vi "RPC Method RouteGuide GetFeature.vi"(3 "error in (no error)":errorcluster, 4 "gRPCid in":T2, 5 "DNL_LabVIEW Object in":refnum<class "RouteGuideImpl.lvclass">) -> (0 "error out":errorcluster, 1 "gRPCid out":T2, 2 "DNL_LabVIEW Object out":refnum<class "RouteGuideImpl.lvclass">)   [LabVIEW 2019, in "UserCode_impl_server.lvlib" / "RouteGuideImpl.lvclass"]
uses:
  RouteGuideImpl.lvclass
  <vilib>/gRPC/LabVIEW gRPC Library/Shared/grpcId.ctl
  Generated_stub_server/RPC Messages/routeguide_Point.ctl
  Generated_stub_server/RPC Service/RouteGuideStub/RouteGuideStub.lvclass
  Generated_stub_server/Generated_stub_server.lvlib
  <vilib>/gRPC/LabVIEW gRPC Library/grpc-lvsupport-release.lvlib
panel:
  in  "?":cluster{"name":string, "location":T1}
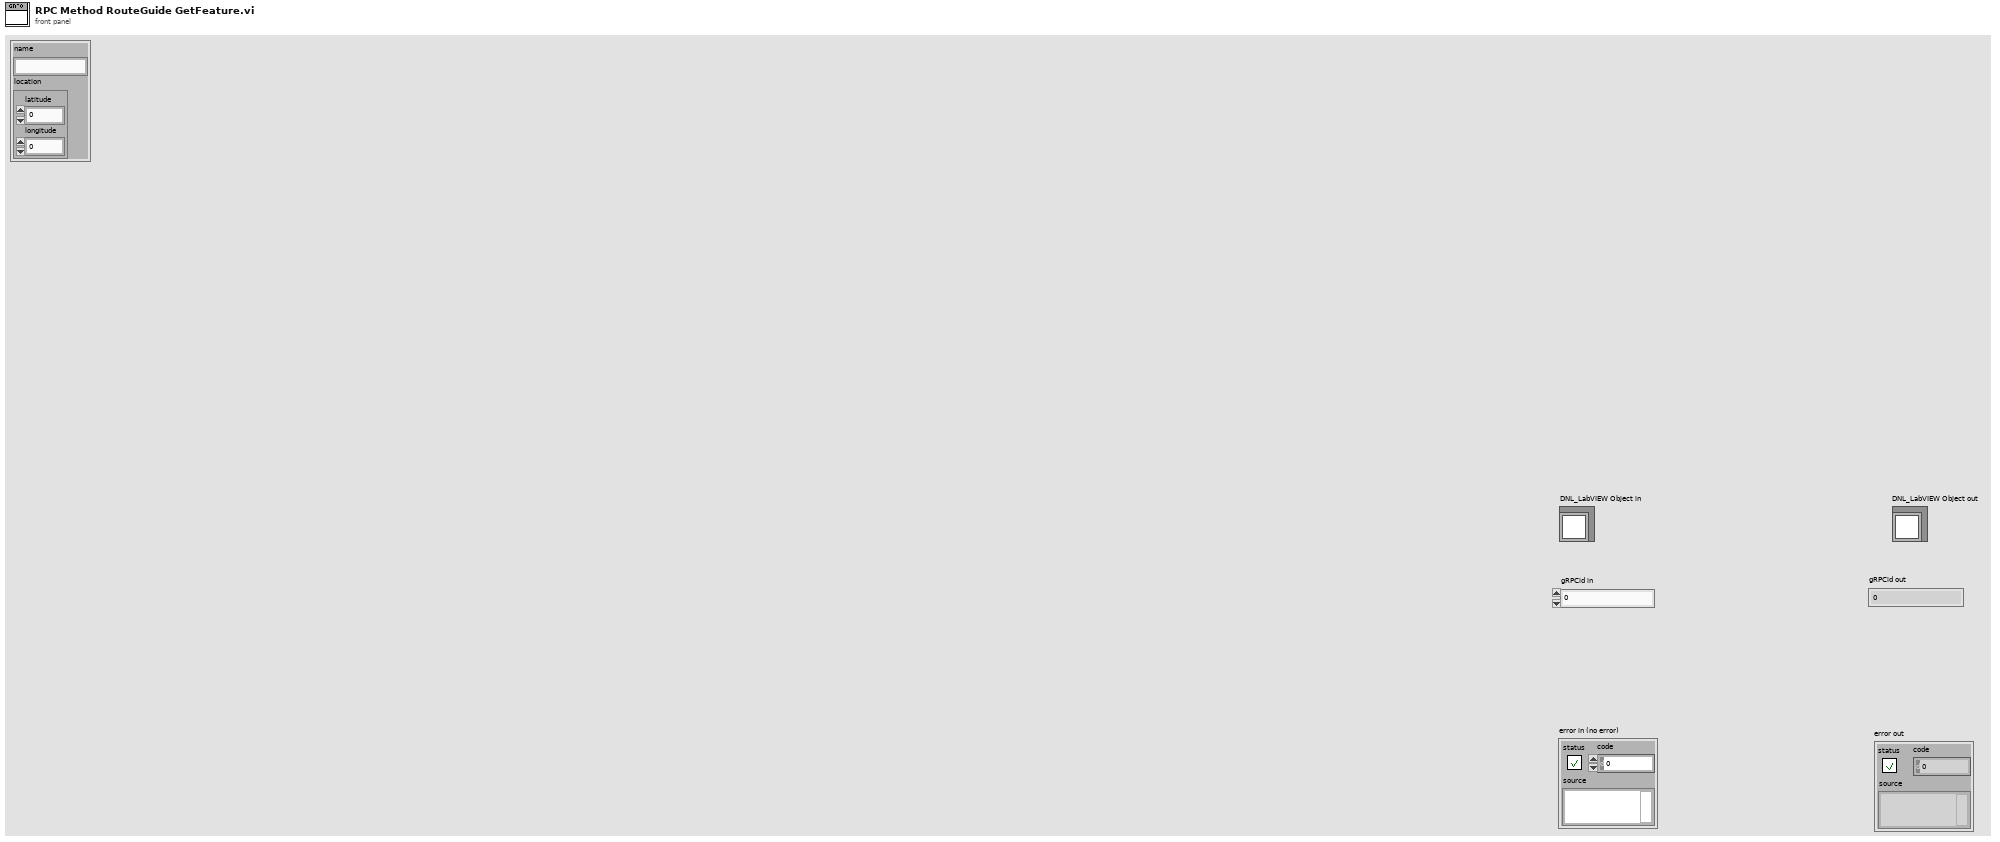
[diagram p1: front panel]
types:
  T1 = typedef "Generated_stub_server.lvlib/routeguide_Point.ctl" = cluster{"latitude":i32, "longitude":i32}
  T2 = typedef "grpc-lvsupport-release.lvlib/grpcId.ctl" = u64
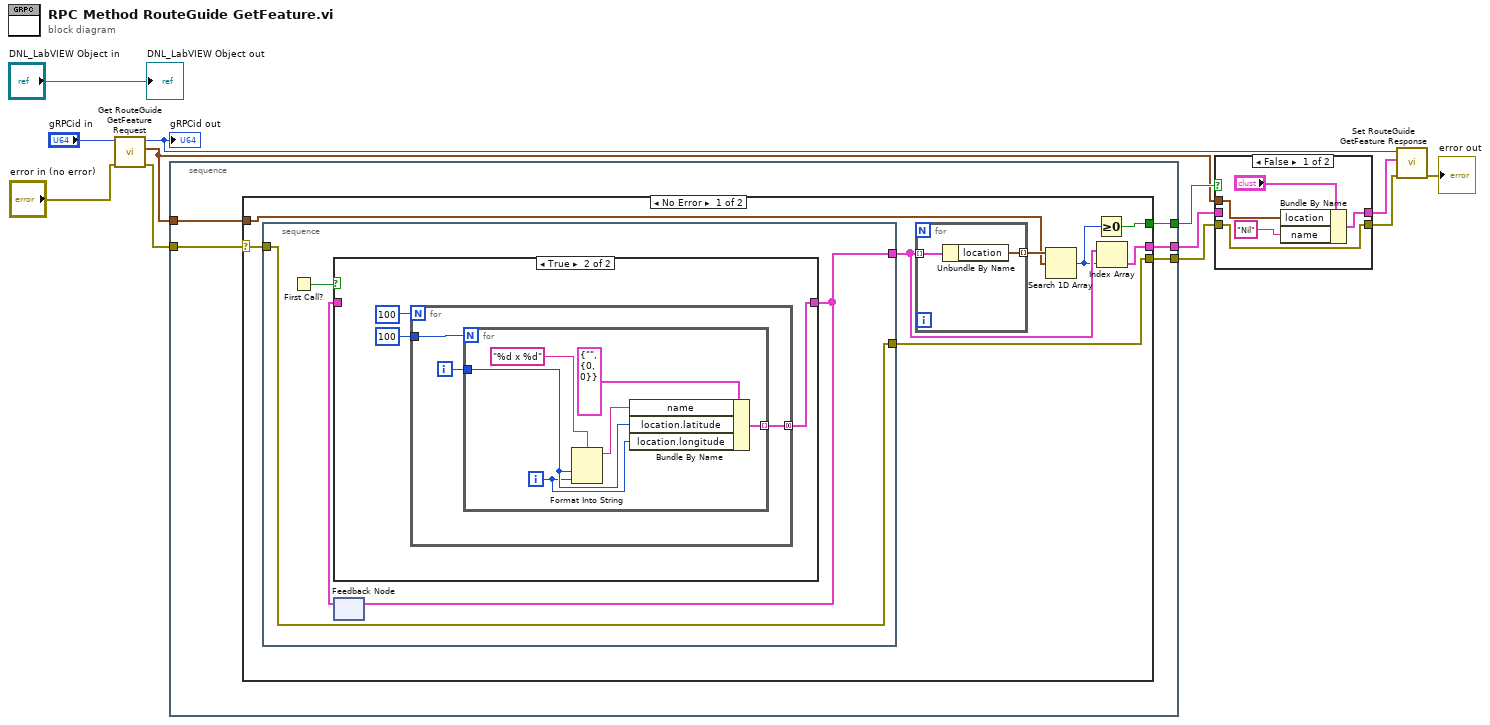
[diagram p0: block diagram]
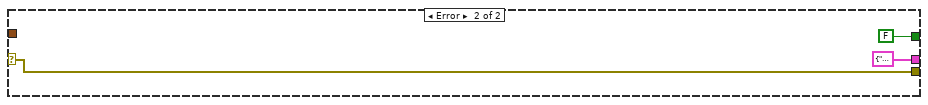
[diagram p3: hidden frame]
diagram:
  n1 = call "Get RouteGuide GetFeature Request.vi"("error in (no error)"="error in (no error)", "gRPCid"="gRPCid in") -> ("error out"=w9:errorcluster, "Message Data"=w8:T1, "gRPCid out"=w2:T2)  [unwired: 7 in]
  "gRPCid out" <- w2
  n2 = stacked-sequence {
    tunnel: [w14] -> w10
    tunnel: [w17] -> w12
    tunnel: [w16] -> w11
    tunnel: w9 -> [w13]
    tunnel: w8 -> [w15]
    frame #0 {
      n3 = case shown="No Error" w13 {
        selector: w13 -> [w25 w47]
        tunnel: [w24 w47] -> w14
        tunnel: w15 -> [w22 _]
        tunnel: [w19 cluster{"name":string, "routeguide_Point":T1} {"name"="", "routeguide_Point"={"latitude"=0, "longitude"=0}} ("routeguide_Feature")] -> w16
        tunnel: [w18 FALSE] -> w17
        frame No Error {
          n4 = stacked-sequence {
            tunnel: [w26] -> w24
            tunnel: [w28] -> w21
            tunnel: w25 -> [w26]
            frame #0 {
              n5 = First Call?() -> (First Call?: T/F=w27:bool)
              n6 = feedback #1() -> (w29:cluster{"name":string, "location":T1}[])  [unwired: 1 in]
              n7 = case shown="True" w27 {
                tunnel: [w30 w31] -> w28
                tunnel: w29 -> [w30 _]
                frame False {
                }
                frame True {
                  n8 = for {
                    N: 100 -> [_]
                    tunnel: [w34] -> w31 mode=concatenating
                    tunnel: 100 -> [w36]
                    i -> [w35]
                    n9 = for {
                      N: w36 -> [_]
                      tunnel: w35 -> [w39]
                      tunnel: [w37] -> w34 mode=indexing
                      i -> [w38]
                      n10 = Format Into String(format string="%d x %d", w39, w38) -> (resulting string=w40:string)  [unwired: 2 in, 1 out]
                      n11 = Bundle By Name(cluster=cluster{"name":string, "location":T1} {"name"="", "location"={"latitude"=0, "longitude"=0}} ("routeguide_Feature"), "name"=w40, "location.latitude"=w39, "location.longitude"=w38) -> (w37:cluster{"name":string, "location":T1})
                    }
                  }
                }
              }
              n12 = feedback-in #1(w28) -> ()
            }
          }
          n13 = for {
            tunnel: w21 -> [w44] mode=indexing
            tunnel: [w43] -> w23 mode=indexing
            n14 = Unbundle By Name(w44) -> ("location"=w43:T1)
          }
          n15 = Search 1D Array(1D array=w23, element=w22) -> (index of element=w20:i32)  [unwired: 1 in]
          n16 = Greater Or Equal To 0?(x=w20) -> (x >= 0?=w18:bool)
          n17 = Index Array(array=w21, index=w20) -> (element=w19:cluster{"name":string, "location":T1})
        }
        frame Error {
        }
      }
    }
  }
  n18 = case shown="False" w12 {
    tunnel: w11 -> [_ w54]
    tunnel: w10 -> [w52 w53]
    tunnel: [w51 w54] -> w7
    tunnel: [w52 w53] -> w6
    tunnel: w8 -> [w50 _]
    frame False {
      n19 = Bundle By Name(cluster="?", "location"=w50, "name"="Nil") -> (w51:cluster{"name":string, "location":T1})
    }
    frame True {
    }
  }
  n20 = call "Set RouteGuide GetFeature Response.vi"("error in (no error)"=w6, "Message Data"=w7, "gRPCid in"=w2) -> ("error out"=→"error out":errorcluster)  [unwired: 8 in]
  "DNL_LabVIEW Object out" <- "DNL_LabVIEW Object in"
